vi "Get Measurement Function.vi"(8 "error in (no error)":errorcluster, 11 "VISA resource name":refnum<visa-resource-name>) -> (0 "error out":errorcluster, 2 "Measurement Function":string, 3 "VISA resource name out":refnum<visa-resource-name>)   [LabVIEW 2021, in "Keithley 2450.lvlib"]
doc: "Gets measurement function on the instrument."
uses:
  Keithley 2450.lvlib
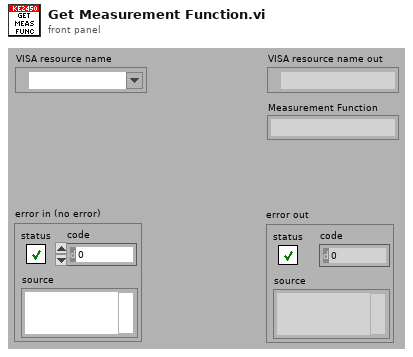
[diagram p1: front panel]
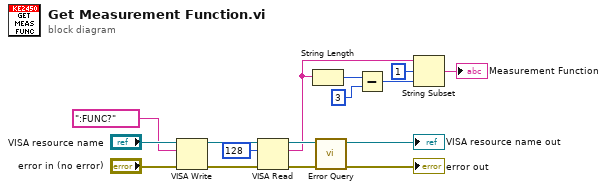
[diagram p0: block diagram]
diagram:
  n1 = VISA Write(VISA resource name="VISA resource name", write buffer=":FUNC?", error in (no error)="error in (no error)") -> (VISA resource name out=w9:refnum<visa-resource-name>, error out=w11:errorcluster)  [unwired: 1 out]
  n2 = VISA Read(VISA resource name=w9, byte count=u32 128, error in (no error)=w11) -> (VISA resource name out=w8:refnum<visa-resource-name>, read buffer=w5:string, error out=w10:errorcluster)  [unwired: 1 out]
  n3 = String Length(string=w5) -> (length=w4:i32)
  n4 = call "Error Query.vi"("error in (no error)"=w10, "VISA resource name"=w8) -> ("error out"=→"error out":errorcluster, "VISA resource name out"=→"VISA resource name out":refnum<visa-resource-name>)  [unwired: 8 out]
  n5 = Subtract(x=w4, y=3) -> (x-y=w3:i32)
  n6 = String Subset(string=w5, offset (0)=1, length (rest)=w3) -> (substring=→"Measurement Function":string)
